vi "FarFiledCamTest.vi"() -> ()   [LabVIEW 2018]
panel:
  out "x-y":u32
  out "1/x":dbl
  in  "停止":bool
  out "error out":errorcluster
  out "通信正常":bool
  out "Image":T1(plugin-control)
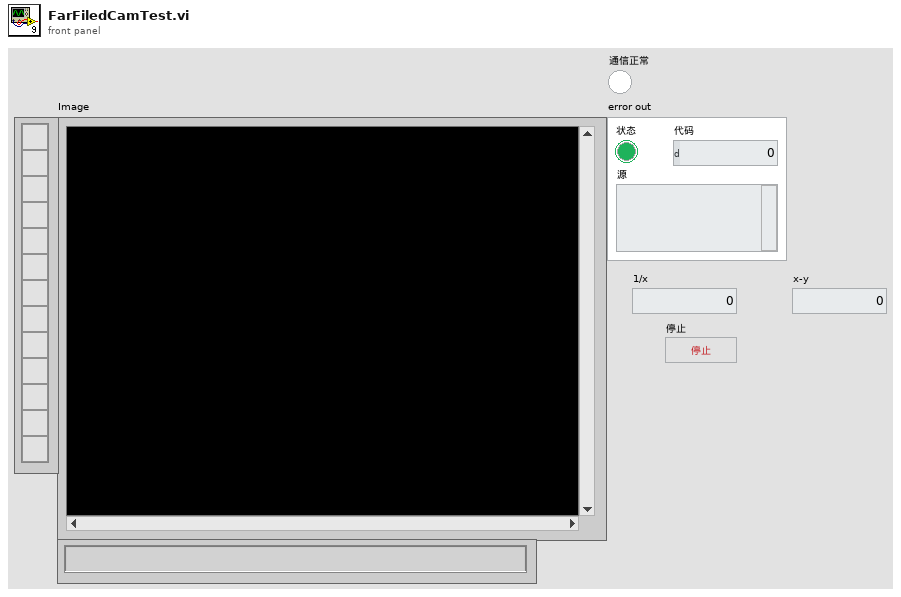
[diagram p1: front panel]
types:
  T1 = typedef "IMAQ Image.ctl" = refnum<image>
  T2 = cluster{"示波器":cluster{"Channel (0:Channel 1)":enum16{"Channel 1", "Channel 2", "Channel 3", "Channel 4"}, "电压范围":dbl, "触发电压":dbl, "时间范围":dbl, " 示波器VISA":refnum<visa-resource-name>, "时间范围 标签":u64, "电压范围 标签":u64, "触发电压 标签":u64, "输入阻抗/Ω":u64}, "光谱仪":cluster{"SpecDataReference":refnum<queue>, "grating center":dbl, "Exposure Time (s)":dbl, "是否进行详细设置":bool, " 开始通信检查":bool, "通信成功？":bool, "波长":dbl}, " 近场相机":cluster{"曝光时间/100us":dbl, "模拟增益":i32, "控制套接字":i32, "IP 地址":string, " 采集套接字":i32, "  版本号":i32, "ImageData":T1, "  增益最大":i32, "  增益最小":i32, " 曝光最大":i32, " 曝光最小":i32, " 帧速":i32, " 同步切换":i32, "  曝光缩放":i32}, " 偏振仪":cluster{"电压范围":u64, "触发电压":u64, "时间范围":u64, "波长范围":enum16{"可见光 400-700nm", "近红外 700-1100nm"}, "可见光偏振测量仪VISA":refnum<visa-resource-name>, "近红外偏振测量仪VISA":refnum<visa-resource-name>}, " 功率计":cluster{"通道":enum16{"Channel 1", "Channel 2"}, "工作波长":u32, "单位":u64, "时间范围":u64, "IP地址":string, "端口":u32}, "能量计":cluster{"通道":enum16{"Channel 1", "Channel 2"}, "工作波长":u32, "单位":u64, "时间范围":u64, "IP地址":string, "端口":u32, "能量计量程":enum16{"200uJ", "20uJ", "2uJ", "200nJ"}}, "电机":cluster{"Channel (0:Channel 1)":enum16{"Channel 1", "Channel 2", "Channel 3", "Channel 4"}, "电压范围":u64, "触发电压":u64, "时间范围":u64}, " 远场相机":cluster{"曝光时间":i32, "模拟增益":i32, "控制套接字":i32, "IP 地址":string, " 采集套接字":i32, "  版本号":i32, "ImageData":T1, "  增益最大":i32, "  增益最小":i32, " 曝光最大":i32, " 曝光最小":i32, " 帧速":i32, " 同步切换":i32, "  曝光缩放":i32, "ImageData B":T1}}
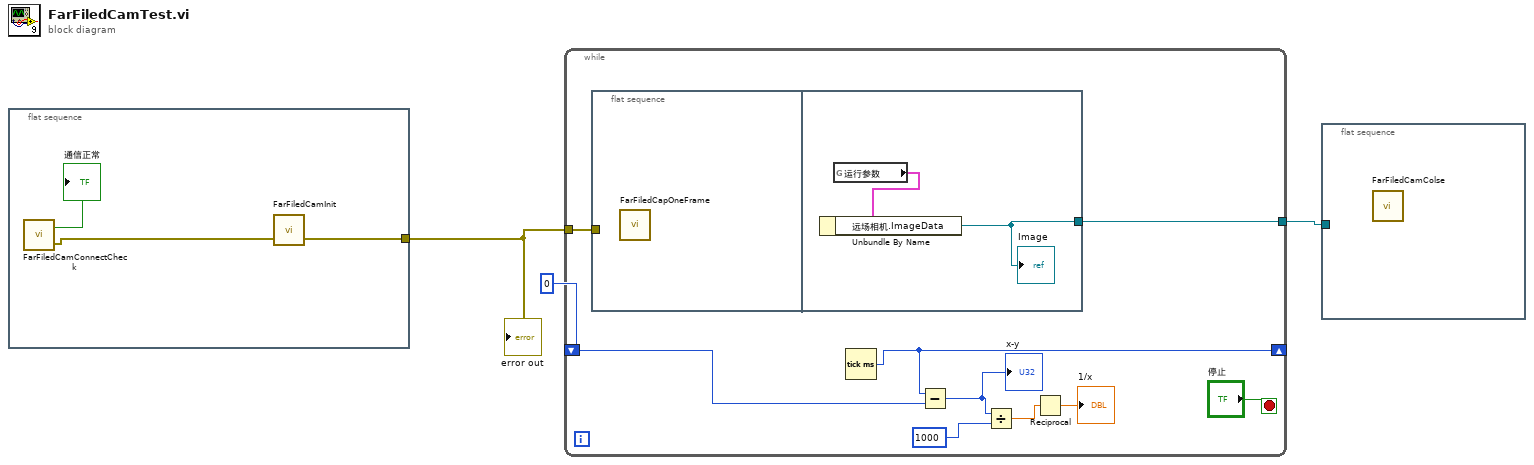
[diagram p0: block diagram]
diagram:
  n1 = flat-sequence {
    tunnel: [w5] -> w3
    frame #0 {
      n2 = call "FarFiledCamConnectCheck.vi"() -> ("error out"=w6:errorcluster, "通信正常"=→"通信正常":bool)  [unwired: 2 in]
      n3 = call "FarFiledCamInit.vi"("error in (no error)"=w6) -> ("error out"=w5:errorcluster)  [unwired: 2 in]
    }
  }
  n4 = while {
    tunnel: w3 -> [w15]
    tunnel: [w14] -> w2
    shift-right: [w12] -> _
    shift-left: u32 0 ("millisecond timer value") -> [w11]
    stop <- "停止" stop-if-true
    n5 = flat-sequence {
      tunnel: w15 -> [_]
      tunnel: [w16] -> w14
      frame #0 {
        n6 = call "FarFiledCapOneFrame.vi"() -> ()  [unwired: 11 in, 1 out]
      }
      frame #1 {
        n7 = global read "参数.vi" "运行参数"() -> (w17:T2)
        n8 = Unbundle By Name(w17) -> ("远场相机.ImageData"=w16:T1)
        "Image" <- w16
      }
    }
    n9 = Tick Count (ms)() -> (millisecond timer value=w12:u32)
    n10 = Subtract(x=w12, y=w11) -> (x-y=w9:u32)
    "x-y" <- w9
    n11 = Divide(x=w9, y=u32 1000) -> (x/y=w7:dbl)
    n12 = Reciprocal(x=w7) -> (1/x=→"1/x":dbl)
  }
  n13 = flat-sequence {
    tunnel: w2 -> [_]
    frame #0 {
      n14 = call "FarFiledCamColse.vi"() -> ()  [unwired: 12 in]
    }
  }
  "error out" <- w3
